vi "Demo_MicrophoneTest - Copy.vi"() -> ()   [LabVIEW 2018]
uses:
  <vilib>/addons/_NISVFA/_Shared subVIs/Controls/svc_DSA Channel Settings.ctl
  <vilib>/addons/_NISVFA/_Shared subVIs/Controls/svc_Engineering Units Text Ring.ctl
  <vilib>/addons/_NISVFA/_Shared subVIs/Controls/svc_Weighting Filter Text Ring.ctl
  <vilib>/addons/_NISVFA/_Shared subVIs/Controls/svc_Channel Info.ctl
  Microfontest/Peiker_Stepped Sweep Settings.ctl
panel:
  in  "Exit":bool
  out "Start":bool
  in  "AI - Response channel":tag="SOUNDACQ/ai1"
  in  "AO channel":tag="SOUNDACQ/ao0"
  in  "FrequencyListFilePath":path=path "D:/Valeo/Micriphone Test/Config/ME79_Limits.csv"
  in  "Response channel Setting":T1={"sensor sensitivity"=1000.0, "engineering units"=1, "dB reference"=1.0, "custom label"="EU", "weighting filter"=0, "pregain"=0.0} {"pregain" format="%.2f"; "weighting filter" items=["Linear", "A-weighting", "B-weighting", "C-weighting", "ITU-R 468-4", "Dolby", "CCITT", "C-message", "Wb", "Wc", "Wd", "We", "Wf", "Wh", "Wj", "Wk", "Wm", "AES17 20 kHz lowpass", "AES17 40 kHz lowpass", "AES17 20 kHz highpass", "AES17 40 kHz highpass"]; "dB reference" format="%^.1e"; "engineering units" items=["custom..."=0, "V"=1, "A"=21, "C"=30, "pC"=31, "s"=32, "-"=29, "Pa"=2, "N"=20, "g"=3, "m/s^2"=4, "m/s"=5, "m"=6, "mm/s"=12, "mm"=13, "micron/s"=14, "micron"=15, "in/s^2"=7, "in/s"=8, "in"=9, "mil/s"=10, "mil"=11, "rad/s^2"=16, "rad/s"=17, "rad"=18, "deg/s^2"=26, "deg/s"=27, "deg"=28, "RPM"=22, "cycle/s^2"=23, "Hz"=24, "cycle"=25, "strain"=19]; "sensor sensitivity" format="%#_5f"}
  in  "Stimulus channel Setting":T1={"sensor sensitivity"=1000.0, "engineering units"=1, "dB reference"=1.0, "custom label"="EU", "weighting filter"=0, "pregain"=0.0} {"pregain" format="%.2f"; "weighting filter" items=["Linear", "A-weighting", "B-weighting", "C-weighting", "ITU-R 468-4", "Dolby", "CCITT", "C-message", "Wb", "Wc", "Wd", "We", "Wf", "Wh", "Wj", "Wk", "Wm", "AES17 20 kHz lowpass", "AES17 40 kHz lowpass", "AES17 20 kHz highpass", "AES17 40 kHz highpass"]; "dB reference" format="%^.1e"; "engineering units" items=["custom..."=0, "V"=1, "A"=21, "C"=30, "pC"=31, "s"=32, "-"=29, "Pa"=2, "N"=20, "g"=3, "m/s^2"=4, "m/s"=5, "m"=6, "mm/s"=12, "mm"=13, "micron/s"=14, "micron"=15, "in/s^2"=7, "in/s"=8, "in"=9, "mil/s"=10, "mil"=11, "rad/s^2"=16, "rad/s"=17, "rad"=18, "deg/s^2"=26, "deg/s"=27, "deg"=28, "RPM"=22, "cycle/s^2"=23, "Hz"=24, "cycle"=25, "strain"=19]; "sensor sensitivity" format="%#_5f"}
  in  "AI - Stimulus channel":tag="SOUNDACQ/ai0"
  in  "Init Amplitude [V]":dbl=1.0
  out "Fundamental-Response":T4(graph)
  out "Response Level":cluster{"frequency":dbl[], "magnitude":dbl[]}(graph)
  out "Stimulus Level":cluster{"frequency":dbl[], "magnitude":dbl[]}(graph)
  in  "Frequency [Hz]":dbl=1000.0
  out "Sensitivity (dBSPL)":dbl
  out "Sensitivity Frequency (Hz)":dbl
  in  "Std_Deviation_Thresold":dbl=0.04 format="%#_13g"
  out "THD-Response":cluster{"frequency":dbl[], "THD":dbl[]}(graph)
  out "THD-Stimulus Level":cluster{"frequency":dbl[], "magnitude":dbl[]}(graph) caption="Stimulus Level"
  in  "THD Frequency":dbl=1000.0
  out "Frequency list Input":T5(array[cluster])=[{"frequency [Hz]"=103.0, "amplitude [V]"=0.09342446715491094}] {"amplitude [V]" format="%.6f"; "frequency [Hz]" format="%.2f"}
  in  "Peiker_Stepped Sweep Settings":T6={"Input Settings"={"IEPE min time to settle [s]"=0.0, "Responce Channel Settings"={"DSA response channel settings"={"coupling"=10045, "enable IEPE excitation"=FALSE, "IEPE current [mA]"=4.0}, "response channel info"={"sensor sensitivity"=1000.0, "engineering units"=1, "dB reference"=1.0, "custom label"="EU", "weighting filter"=0, "pregain"=0.0}, "AI response settings"={"response channel"="SOUNDACQ/ai1", "max value [V]"=10.0, "min value [V]"=-10.0, "terminal configuration"=-1}}, "Stimulus Channel Settings"={"AI stimulus settings"={"stimulus channel"="SOUNDACQ/ai0", "max value [V]"=10.0, "min value [V]"=-10.0, "terminal configuration"=-1}, "DSA stimulus channel settings"={"coupling"=10045, "enable IEPE excitation"=FALSE, "IEPE current [mA]"=4.0}, "stimulus channel info"={"sensor sensitivity"=11.4, "engineering units"=2, "dB reference"=2e-05, "custom label"="EU", "weighting filter"=0, "pregain"=0.0}}}, "Output Settings"={"AO source settings"={"excitation channel"="SOUNDACQ/ao0", "max value [V]"=10.0, "min value [V]"=-10.0, "terminal configuration"=-1}}} {"Output Settings"."AO source settings"."terminal configuration" items=["Default"=-1, "RSE"=10083, "Differential"=10106, "Pseudodifferential"=12529]; "Output Settings"."AO source settings"."min value [V]" format="%0.2f"; "Output Settings"."AO source settings"."max value [V]" format="%0.2f"; "Input Settings"."Stimulus Channel Settings"."stimulus channel info"."pregain" format="%.2f"; "Input Settings"."Stimulus Channel Settings"."stimulus channel info"."weighting filter" items=["Linear", "A-weighting", "B-weighting", "C-weighting", "ITU-R 468-4", "Dolby", "CCITT", "C-message", "Wb", "Wc", "Wd", "We", "Wf", "Wh", "Wj", "Wk", "Wm", "AES17 20 kHz lowpass", "AES17 40 kHz lowpass", "AES17 20 kHz highpass", "AES17 40 kHz highpass"]; "Input Settings"."Stimulus Channel Settings"."stimulus channel info"."dB reference" format="%^.1e"; "Input Settings"."Stimulus Channel Settings"."stimulus channel info"."engineering units" items=["custom..."=0, "V"=1, "A"=21, "C"=30, "pC"=31, "s"=32, "-"=29, "Pa"=2, "N"=20, "g"=3, "m/s^2"=4, "m/s"=5, "m"=6, "mm/s"=12, "mm"=13, "micron/s"=14, "micron"=15, "in/s^2"=7, "in/s"=8, "in"=9, "mil/s"=10, "mil"=11, "rad/s^2"=16, "rad/s"=17, "rad"=18, "deg/s^2"=26, "deg/s"=27, "deg"=28, "RPM"=22, "cycle/s^2"=23, "Hz"=24, "cycle"=25, "strain"=19]; "Input Settings"."Stimulus Channel Settings"."stimulus channel info"."sensor sensitivity" format="%#_5f"; "Input Settings"."Stimulus Channel Settings"."DSA stimulus channel settings"."IEPE current [mA]" format="%.1f"; "Input Settings"."Stimulus Channel Settings"."DSA stimulus channel settings"."coupling" items=["AC"=10045, "DC"=10050, "GND"=10066]; "Input Settings"."Stimulus Channel Settings"."AI stimulus settings"."terminal configuration" items=["Default"=-1, "RSE"=10083, "NRSE"=10078, "Differential"=10106, "Pseudodifferential"=12529]; "Input Settings"."Stimulus Channel Settings"."AI stimulus settings"."min value [V]" format="%.2f"; "Input Settings"."Stimulus Channel Settings"."AI stimulus settings"."max value [V]" format="%.2f"; "Input Settings"."Responce Channel Settings"."AI response settings"."terminal configuration" items=["Default"=-1, "RSE"=10083, "NRSE"=10078, "Differential"=10106, "Pseudodifferential"=12529]; "Input Settings"."Responce Channel Settings"."AI response settings"."min value [V]" format="%.2f"; "Input Settings"."Responce Channel Settings"."AI response settings"."max value [V]" format="%.2f"; "Input Settings"."Responce Channel Settings"."response channel info"."pregain" format="%.2f"; "Input Settings"."Responce Channel Settings"."response channel info"."weighting filter" items=["Linear", "A-weighting", "B-weighting", "C-weighting", "ITU-R 468-4", "Dolby", "CCITT", "C-message", "Wb", "Wc", "Wd", "We", "Wf", "Wh", "Wj", "Wk", "Wm", "AES17 20 kHz lowpass", "AES17 40 kHz lowpass", "AES17 20 kHz highpass", "AES17 40 kHz highpass"]; "Input Settings"."Responce Channel Settings"."response channel info"."dB reference" format="%^.1e"; "Input Settings"."Responce Channel Settings"."response channel info"."engineering units" items=["custom..."=0, "V"=1, "A"=21, "C"=30, "pC"=31, "s"=32, "-"=29, "Pa"=2, "N"=20, "g"=3, "m/s^2"=4, "m/s"=5, "m"=6, "mm/s"=12, "mm"=13, "micron/s"=14, "micron"=15, "in/s^2"=7, "in/s"=8, "in"=9, "mil/s"=10, "mil"=11, "rad/s^2"=16, "rad/s"=17, "rad"=18, "deg/s^2"=26, "deg/s"=27, "deg"=28, "RPM"=22, "cycle/s^2"=23, "Hz"=24, "cycle"=25, "strain"=19]; "Input Settings"."Responce Channel Settings"."response channel info"."sensor sensitivity" format="%#_5f"; "Input Settings"."Responce Channel Settings"."DSA response channel settings"."IEPE current [mA]" format="%.1f"; "Input Settings"."Responce Channel Settings"."DSA response channel settings"."coupling" items=["AC"=10045, "DC"=10050, "GND"=10066]; "Input Settings"."IEPE min time to settle [s]" format="%.1f"}
  out "Init Frequency List":T5(array[cluster])
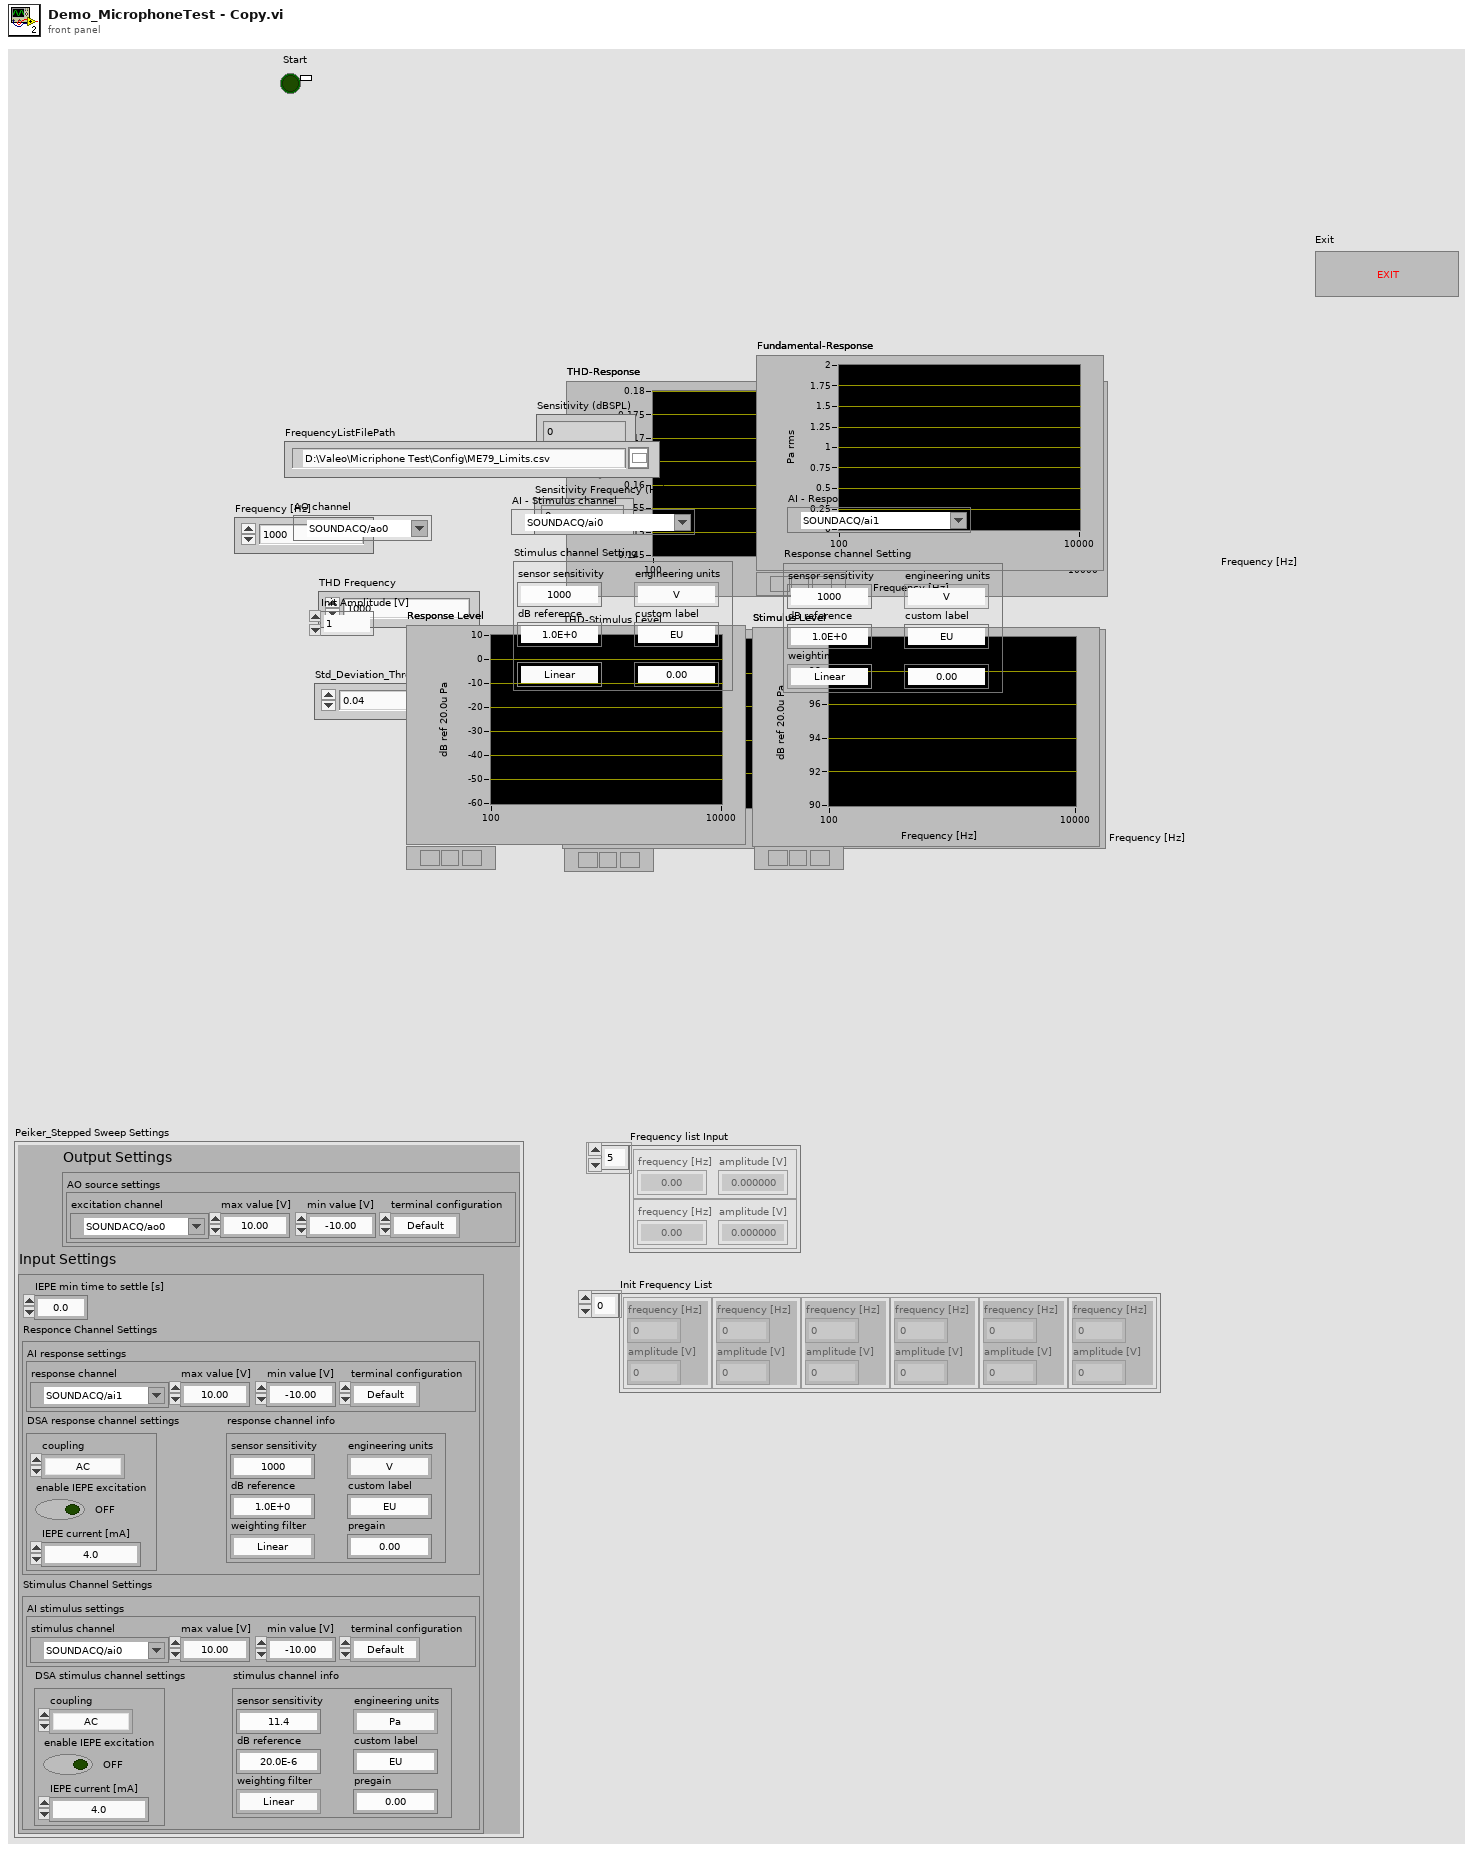
[diagram p1: front panel]
types:
  T1 = typedef "svc_Channel Info.ctl" = cluster{"sensor sensitivity":dbl, "engineering units":T2, "dB reference":dbl, "custom label":string, "weighting filter":T3, "pregain":dbl}
  T2 = typedef "svc_Engineering Units Text Ring.ctl" = u16
  T3 = typedef "svc_Weighting Filter Text Ring.ctl" = u16
  T4 = cluster{"frequency [Hz]":dbl[], "amplitude":dbl[]}
  T5 = cluster{"frequency [Hz]":dbl, "amplitude [V]":dbl}[]
  T6 = typedef "Peiker_Stepped Sweep Settings.ctl" = cluster{"Input Settings":cluster{"IEPE min time to settle [s]":dbl, "Responce Channel Settings":cluster{"DSA response channel settings":T7, "response channel info":T1, "AI response settings":cluster{"response channel":tag, "max value [V]":dbl, "min value [V]":dbl, "terminal configuration":i32}}, "Stimulus Channel Settings":cluster{"AI stimulus settings":cluster{"stimulus channel":tag, "max value [V]":dbl, "min value [V]":dbl, "terminal configuration":i32}, "DSA stimulus channel settings":T7, "stimulus channel info":T1}}, "Output Settings":cluster{"AO source settings":cluster{"excitation channel":tag, "max value [V]":dbl, "min value [V]":dbl, "terminal configuration":i32}}}
  T7 = typedef "svc_DSA Channel Settings.ctl" = cluster{"coupling":i32, "enable IEPE excitation":bool, "IEPE current [mA]":dbl}
  T8 = cluster{"frequency [Hz]":dbl, "amplitude [V]":dbl}
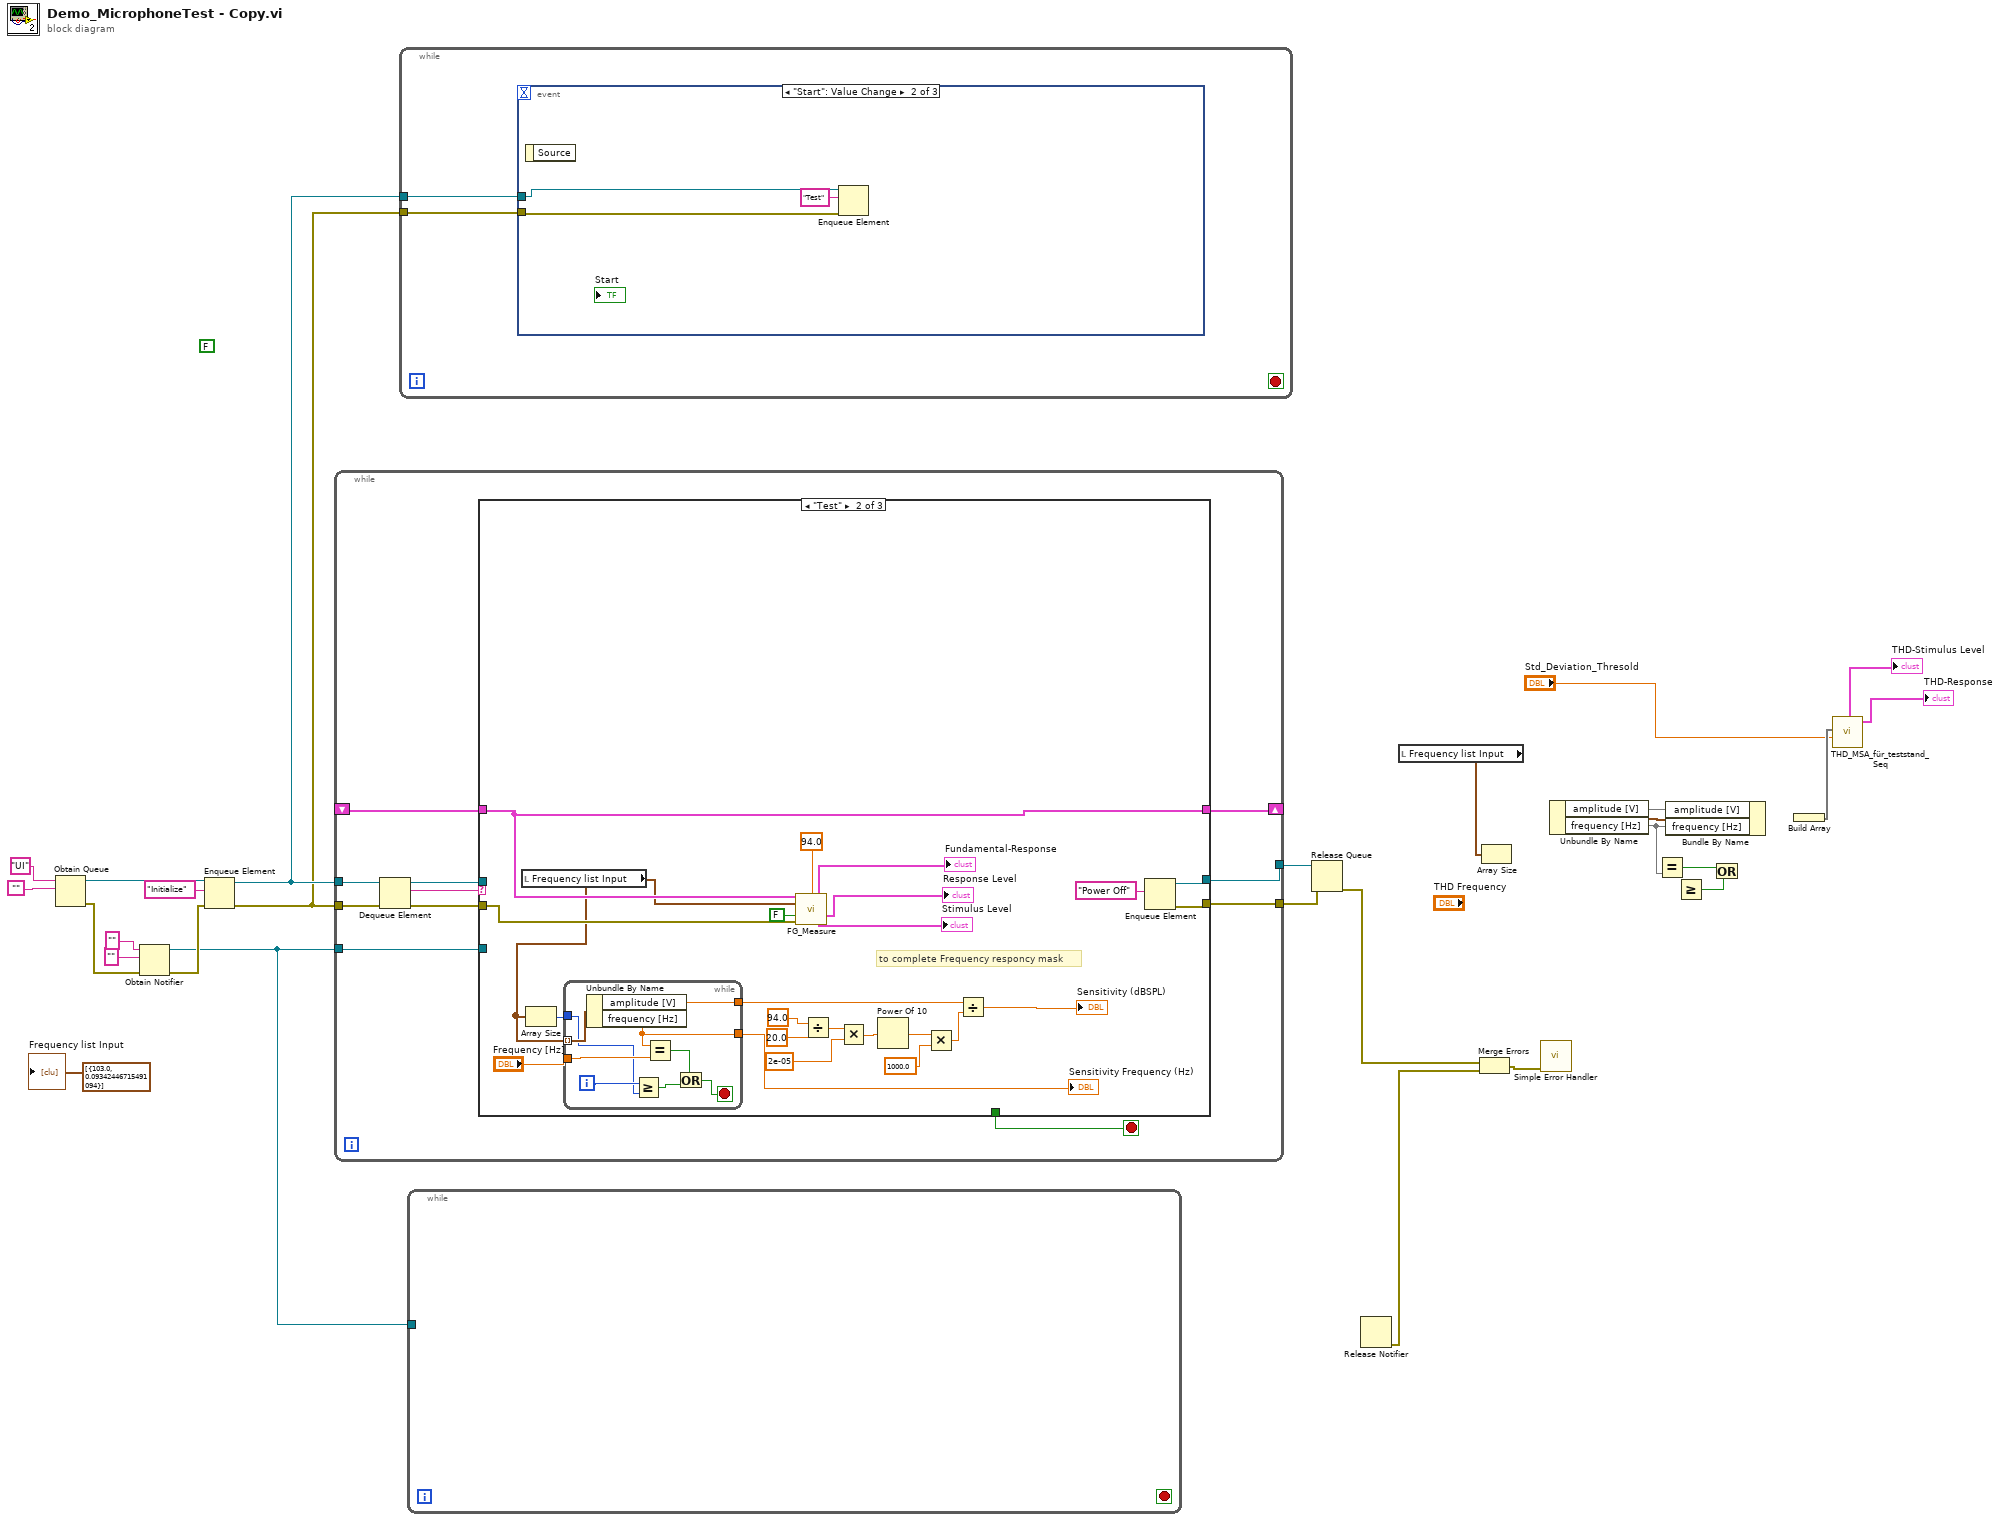
[diagram p0: block diagram]
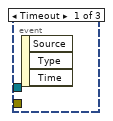
[diagram p2: hidden frame]
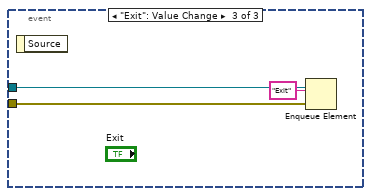
[diagram p3: hidden frame]
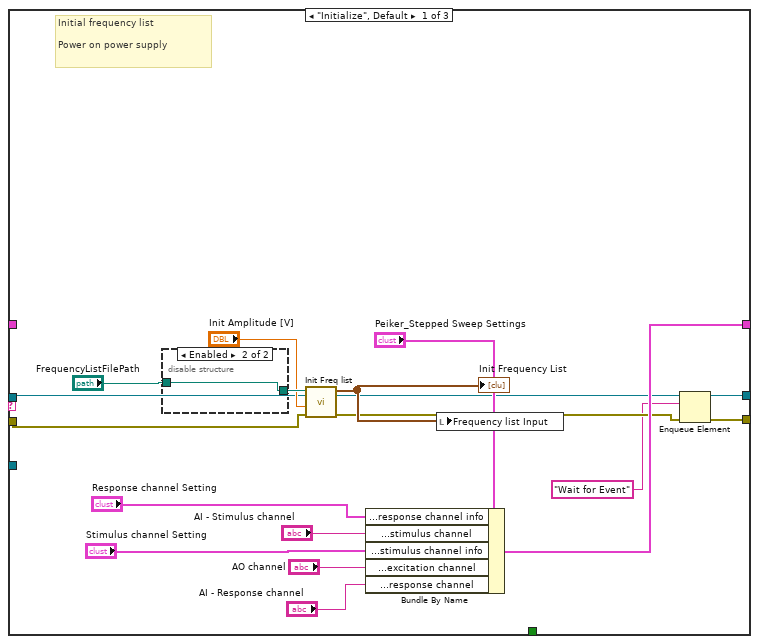
[diagram p4: hidden frame]
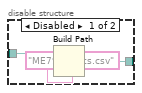
[diagram p5: hidden frame]
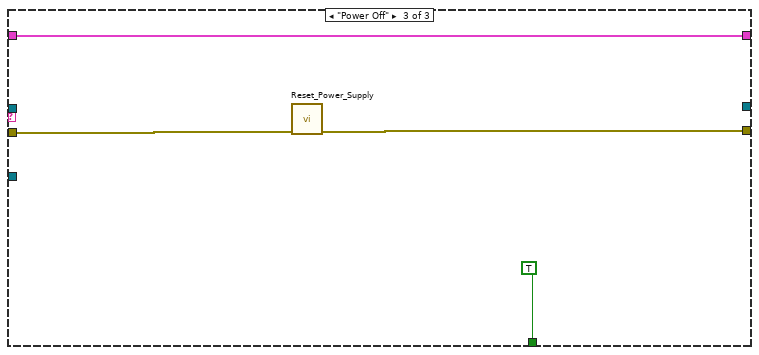
[diagram p6: hidden frame]
diagram:
  (unwired) FALSE ("Start")
  n1 = Obtain Queue(name (unnamed)="UI", element data type="") -> (queue out=w34:refnum<queue>, error out=w25:errorcluster)  [unwired: 3 in, 1 out]
  n2 = Obtain Notifier(name (unnamed)="", notification data type="", error in (no error)=w25) -> (notifier out=w20:refnum<notifier>, error out=w22:errorcluster)  [unwired: 1 in, 1 out]
  n3 = Enqueue Element(queue=w34, element="Initialize", error in (no error)=w22) -> (queue out=w2:refnum<queue>, error out=w1:errorcluster)  [unwired: 1 in, 1 out]
  n4 = while {
    tunnel: w1 -> [w45]
    tunnel: w2 -> [w44]
    shift-right: [w38] -> _
    shift-left: _ -> [w37]
    tunnel: [w40] -> w32
    tunnel: [w35] -> w31
    tunnel: w20 -> [w36]
    stop <- w41 stop-if-true
    n5 = Dequeue Element(queue=w44, error in (no error)=w45) -> (queue out=w39:refnum<queue>, element=w43:string, error out=w42:errorcluster)  [unwired: 1 in, 1 out]
    n6 = case shown="\"Test\"" w43 {
      tunnel: w42 -> [w61 w89 w102]
      tunnel: w39 -> [w47 _ _]
      tunnel: [_ _ TRUE] -> w41
      tunnel: [w49 w69 w101] -> w40
      tunnel: [w58 w85 w100] -> w38
      tunnel: w37 -> [_ w85 w100]
      tunnel: w36 -> [_ _ _]
      tunnel: [w48 w68 _] -> w35
      frame "Initialize", Default {
        # "Initial frequency list\n\nPower on power supply"
        n7 = disable-structure shown="Enabled" {
          disable-tunnel: [w64 w66] -> w62
          disable-tunnel: "FrequencyListFilePath" -> [w63 w66]
          frame Disabled {
            n8 = Build Path(base path=w63, name or relative path="ME79_Limits.csv") -> (appended path=w64:path)
          }
          frame Enabled {
          }
        }
        n9 = call "Init Freq list.vi"("FrequencyListFile path"=w62, "Init Amplitude [V]"="Init Amplitude [V]", "error in (no error)"=w61) -> ("Frequency List"=w54:T5, "error out"=w50:errorcluster)  [unwired: 6 in]
        "Init Frequency List" <- w54
        n10 = Bundle By Name(cluster="Peiker_Stepped Sweep Settings", "Input Settings.Responce Channel Settings.response channel info"="Response channel Setting", "Input Settings.Stimulus Channel Settings.AI stimulus settings.stimulus channel"="AI - Stimulus channel", "Input Settings.Stimulus Channel Settings.stimulus channel info"="Stimulus channel Setting", "Output Settings.AO source settings.excitation channel"="AO channel", "Input Settings.Responce Channel Settings.AI response settings.response channel"="AI - Response channel") -> (w58:T6)
        n11 = local write "Frequency list Input"(w54) -> ()
        n12 = Enqueue Element(queue=w47, element="Wait for Event", error in (no error)=w50) -> (queue out=w48:refnum<queue>, error out=w49:errorcluster)  [unwired: 1 in, 1 out]
      }
      frame "Test" {
        # "to complete Frequency responcy mask"
        n13 = local read "Frequency list Input"() -> (w71:T5)
        n14 = Array Size(array=w71) -> (size(s)=w70:i32)
        n15 = while {
          tunnel: w71 -> [w99] mode=indexing
          tunnel: "Frequency [Hz]" -> [w98]
          tunnel: [w97] -> w82
          tunnel: [w96] -> w72
          tunnel: w70 -> [w92]
          i -> [w93]
          stop <- w95 stop-if-true
          n16 = Unbundle By Name(w99) -> ("amplitude [V]"=w97:dbl, "frequency [Hz]"=w96:dbl)
          n17 = Greater Or Equal?(x=w93, y=w92) -> (x >= y?=w91:bool)
          n18 = Equal?(x=w96, y=w98) -> (x = y?=w94:bool)
          n19 = Or(x=w94, y=w91) -> (x .or. y?=w95:bool)
        }
        "Sensitivity Frequency (Hz)" <- w72
        n20 = call "FG_Measure.vi"("Peiker_Stepped Sweep Settings"=w85, "FrequencyList Output Level (dBSPL)"=94.0, "frequency list Input"=w71, "true=mehrfach Messen"=FALSE ("true = measure several times"), "error in (no error)"=w89) -> ("Fundamental-Response"=→"Fundamental-Response":T4, "Response Level"=→"Response Level":cluster{"frequency":dbl[], "magnitude":dbl[]}, "Stimulus Level"=→"Stimulus Level":cluster{"frequency":dbl[], "magnitude":dbl[]})  [unwired: 5 in, 3 out]
        n21 = Divide(x=94.0, y=20.0) -> (x/y=w79:dbl)
        n22 = Multiply(x=w79, y=2e-05) -> (x*y=w77:dbl)
        n23 = Power Of 10(x=w77) -> (10^x=w76:dbl)
        n24 = Multiply(x=w76, y=1000.0) -> (x*y=w74:dbl)
        n25 = Divide(x=w82, y=w74) -> (x/y=→"Sensitivity (dBSPL)":dbl)
        n26 = Enqueue Element(element="Power Off") -> (queue out=w68:refnum<queue>, error out=w69:errorcluster)  [unwired: 3 in, 1 out]
      }
      frame "Power Off" {
        n27 = call "Reset_Power_Supply.vi"("error in (no error)"=w102) -> ("error out"=w101:errorcluster)  [unwired: 10 in]
      }
    }
  }
  n28 = while {
    tunnel: w2 -> [w105]
    tunnel: w1 -> [w104]
    stop <- _ stop-if-true
    n29 = event shown="[1] \"Start\": Value Change" {
      selector: _ -> [_ _ _]
      dyn-events: _ -> [_ _ _]
      timeout: _ -> [_ _ _]
      tunnel: w105 -> [_ w108 w111]
      tunnel: w104 -> [_ w107 w110]
      event Timeout {
        n30 = event-data() -> ()  [unwired: 1 in, 3 out]
      }
      event "Start": Value Change {
        n31 = event-data() -> ()  [unwired: 1 in, 1 out]
        n32 = Enqueue Element(queue=w108, element="Test", error in (no error)=w107) -> ()  [unwired: 1 in, 3 out]
      }
      event "Exit": Value Change {
        n33 = event-data() -> ()  [unwired: 1 in, 1 out]
        n34 = Enqueue Element(queue=w111, element="Exit", error in (no error)=w110) -> ()  [unwired: 1 in, 3 out]
      }
    }
  }
  n35 = while {
    tunnel: w20 -> [_]
    stop <- _ stop-if-true
  }
  n36 = Release Queue(queue=w31, error in (no error)=w32) -> (error out=w27:errorcluster)  [unwired: 1 in, 2 out]
  n37 = Release Notifier() -> (error out=w21:errorcluster)  [unwired: 3 in, 2 out]
  n38 = local read "Frequency list Input"() -> (w10:T5)
  n39 = Merge Errors(w27, w21) -> (w26:errorcluster)
  n40 = Array Size(array=w10) -> (size(s)=w11:i32)
  n41 = call <vilib>:"Simple Error Handler.vi"("error in (no error)"=w26) -> ()  [unwired: 4 in, 5 out]
  n42 = Unbundle By Name() -> (w15:T8, "amplitude [V]"=w14, "frequency [Hz]"=w13)
  n43 = Equal?(y=w13) -> (x=w12:dbl, x = y?=w17:bool)
  n44 = Bundle By Name(cluster=w15, "amplitude [V]"=w14, "frequency [Hz]"=w13) -> ()  [unwired: 1 out]
  n45 = Greater Or Equal?() -> (x=w18:dbl, y=w19:dbl, x >= y?=w16:bool)
  n46 = Or(x=w17, y=w16) -> ()  [unwired: 1 out]
  n47 = Build Array() -> (w9:void[])  [unwired: 1 in]
  n48 = call "THD_MSA_für_teststand_Seq.vi"("Std_Deviation_Thresold"="Std_Deviation_Thresold", "frequency list Input"=w9) -> ("Stimulus Level"=→"THD-Stimulus Level":cluster{"frequency":dbl[], "magnitude":dbl[]}, "THD-Response"=→"THD-Response":cluster{"frequency":dbl[], "THD":dbl[]}, "error in"=w4:errorcluster, "Peiker_Stepped Sweep Settings"=w7:T6)  [unwired: 5 in, 1 out]
  "Frequency list Input" <- T5 [{"frequency [Hz]"=103.0, "amplitude [V]"=0.09342446715491094}] ("frequency list Input")
